vi "GetXYGraphReference.vi"(8 "error in":errorcluster, 11 "XYGraph in":refnum<class "XYGraph.lvclass">) -> (0 "error out":errorcluster, 1 "XYGraph reference":refnum<vi>, 3 "XYGraph out":refnum<class "XYGraph.lvclass">)   [LabVIEW 2014, in "XYGraph.lvclass"]
uses:
  XYGraph.lvclass
  Generic/Generic.lvclass
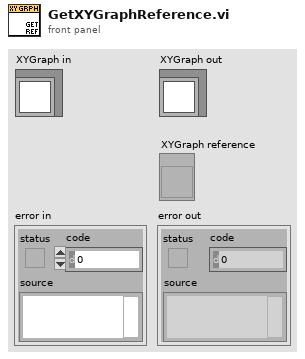
[diagram p1: front panel]
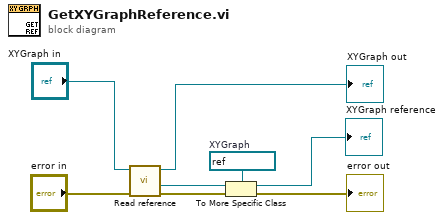
[diagram p0: block diagram]
diagram:
  w5 = refnum<vi> refnum  # XYGraph
  n1 = call "Read reference.vi"("error in"="error in", "GObject in"="XYGraph in") -> ("error out"=w6:errorcluster, "reference"=w7:refnum<vi>, "GObject out"=→"XYGraph out":refnum<class "XYGraph.lvclass">)  [unwired: 5 in]
  n2 = To More Specific Class(target class=w5, reference=w7, error in=w6) -> (specific class reference=→"XYGraph reference":refnum<vi>, error out=→"error out":errorcluster)
